vi "XIPIN_Ultrascale_FPGA_Gen3_Integrated_Block_for_PCI_Express_4_1.vi"   [LabVIEW 2017]
doc: "The Xilinx UltraScale Gen3 Integrated Block for PCI Express (1-lane, 2-lane, 4-lane, and 8-lane) in conjunction with flexible UltraScale architectural features such as integrated GTs (Gigabit Transceivers) and BRAM (Block RAMs) are used to implement a PCI Express Base Specification v3.1 compliant PCI Express devices.\n------------------------------------\n<b>Need License</b> : No\n<b>Interface</b> : AXI4-Stream"
uses:
  <vilib>/rvi/XilinxIP/XIPIN_XNode/niFpgaXIPIN.xnode
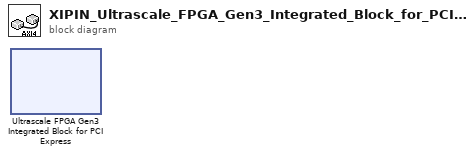
[diagram p0: block diagram]
diagram:
  n1 = xnode ("Ultrascale FPGA Gen3 Integrated Block for PCI Express")() -> ()
